vi "Textanzeige.vi"(9 "Param Text":T1, 11 "Bild":picture) -> (3 "Bild neu":picture)   [LabVIEW 2020, in "Anlagenuebersicht.lvlib" / "VisBx Anzeige.lvlib"]
uses:
  VisBx Anzeige.lvlib
  VisParameter/Param Text.ctl
  VisParameter/VisPunkt.ctl
  VisParameter/VisParam-Typdef.lvlib
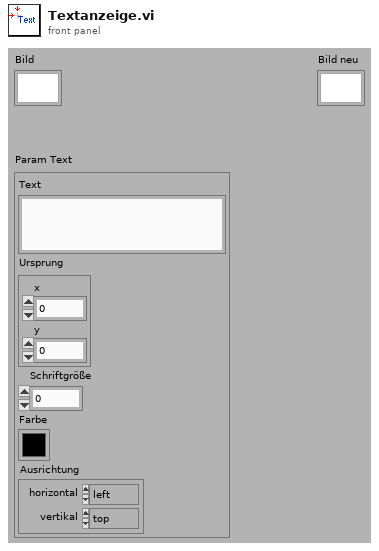
[diagram p1: front panel]
types:
  T1 = typedef "VisParam-Typdef.lvlib/Param Text.ctl" = cluster{"Text":string, "Ursprung":T2, "Schriftgröße":i16, "Farbe":u32, "Ausrichtung":cluster{"horizontal":enum16{"left", "center", "right"}, "vertical":enum16{"top", "center", "bottom"}}}
  T2 = typedef "VisParam-Typdef.lvlib/VisPunkt.ctl" = cluster{"x":i16, "y":i16}
  T3 = cluster{"Font Name:":string, "Size":i16, "Strikeout?":bool, "Italic?":bool, "Underline?":bool, "Outline?":bool, "Shadow?":bool, "Bold?":bool}
  T4 = enum16{"User-specified Font", "Application Font", "System Font", "Dialog Font"}
  T5 = cluster{"horizontal":enum16{"left", "center", "right"}, "vertical":enum16{"top", "center", "bottom"}}
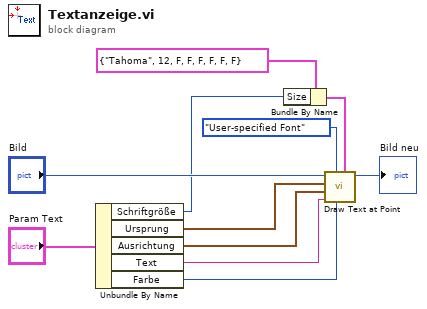
[diagram p0: block diagram]
diagram:
  n1 = Unbundle By Name("Param Text") -> ("Schriftgröße"=w1:i16, "Ursprung"=w8:T2, "Ausrichtung"=w7:T5, "Text"=w6:string, "Farbe"=w5:u32)
  n2 = Bundle By Name(cluster=T3 {"Font Name:"="Tahoma", "Size"=12, "Strikeout?"=FALSE, "Italic?"=FALSE, "Underline?"=FALSE, "Outline?"=FALSE, "Shadow?"=FALSE, "Bold?"=FALSE} ("[user-specified font]"), "Size"=w1) -> (w3:T3)
  n3 = call <vilib>:"Draw Text at Point.vi"("[user-specified font]"=w3, "text color(black)"=w5, "desired font(Application)"=T4."User-specified Font", "text"=w6, "alignment(left, top)"=w7, "origin"=w8, "picture"="Bild") -> ("new picture"=→"Bild neu":picture)  [unwired: 2 in, 2 out]
